vi "updateTCPEvnts.vi"(8 "error in (no error)":errorcluster, 11 "MonoCommunicator in":refnum<class "MonoCommunicator.lvclass">) -> (0 "error out":errorcluster, 3 "MonoCommunicator out":refnum<class "MonoCommunicator.lvclass">)   [LabVIEW 2016, in "MonoCommunicator.lvclass"]
uses:
  MonoCommunicator.lvclass
  MonoCommunicator.lvclass/MonoCommunicator.ctl
  MonoPubSubData/MonoPubSubData.lvclass/MonoPubSubData.ctl
  ts_labview_tcp/TCPCommunicator/TCPCommunicator.lvclass/TCPCommunicator.ctl
  ts_labview_tcp/TCPComEvents/TCPComEvents.lvclass/TCPComEvents.ctl
  ts_labview_tcp/TCPServer/TCPServer.lvclass
  C:/Users/ComputerAdmin/Documents/ts_monochromator_windows/ts_labview_tcp/TCPCommunicator/TCPCommunicator.lvclass
  MonoPubSubData/MonoPubSubData.lvclass
  ts_labview_tcp/TCPComEvents/TCPComEvents.lvclass
  ts_labview_tcp/TCPCommunicator/TCPCommunicator.lvclass
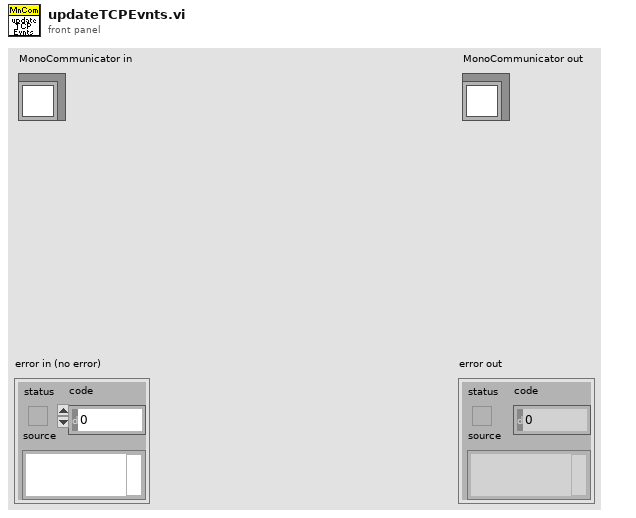
[diagram p1: front panel]
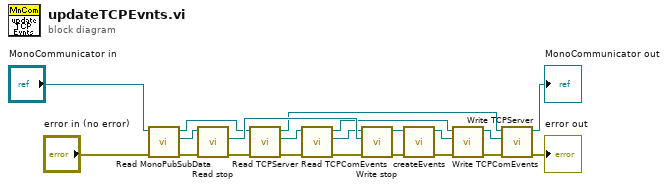
[diagram p0: block diagram]
diagram:
  n1 = call "Read MonoPubSubData.vi"("error in (no error)"="error in (no error)", "MonoCommunicator in"="MonoCommunicator in") -> ("error out"=w7:errorcluster, "MonoPubSubData.lvclass"=w19:refnum<class "MonoPubSubData.lvclass">, "MonoCommunicator out"=w17:refnum<class "MonoCommunicator.lvclass">)  [unwired: 7 in]
  n2 = call "Read stop.vi"("error in (no error)"=w7, "MonoPubSubData in"=w19) -> ("error out"=w8:errorcluster, "stop"=w18:refnum<user-event>)  [unwired: 7 in, 1 out]
  n3 = call "Read TCPServer.vi"("error in (no error)"=w8, "MonoCommunicator in"=w17) -> ("error out"=w16:errorcluster, "TCPServer.lvclass"=w15:refnum<class "TCPServer.lvclass">, "MonoCommunicator out"=w14:refnum<class "MonoCommunicator.lvclass">)  [unwired: 7 in]
  n4 = call "Read TCPComEvents.vi"("error in (no error)"=w16, "TCPCommunicator in"=w15) -> ("error out"=w5:errorcluster, "TCPComEvents.lvclass"=w12:refnum<class "TCPComEvents.lvclass">, "TCPCommunicator out"=w13:refnum<class "TCPServer.lvclass">)  [unwired: 7 in]
  n5 = call "Write stop.vi"("error in (no error)"=w5, "stop"=w18, "TCPComEvents in"=w12) -> ("error out"=w3:errorcluster, "TCPComEvents out"=w4:refnum<class "TCPComEvents.lvclass">)  [unwired: 7 in]
  n6 = call "createEvents.vi"("error in (no error)"=w3, "TCPComEvents in"=w4) -> ("error out"=w2:errorcluster, "TCPComEvents out"=w1:refnum<class "TCPComEvents.lvclass">)  [unwired: 8 in]
  n7 = call "Write TCPComEvents.vi"("error in (no error)"=w2, "TCPComEvents.lvclass"=w1, "TCPCommunicator in"=w13) -> ("error out"=w11:errorcluster, "TCPCommunicator out"=w21:refnum<class "TCPServer.lvclass">)  [unwired: 7 in]
  n8 = call "Write TCPServer.vi"("error in (no error)"=w11, "TCPServer.lvclass"=w21, "MonoCommunicator in"=w14) -> ("error out"=→"error out":errorcluster, "MonoCommunicator out"=→"MonoCommunicator out":refnum<class "MonoCommunicator.lvclass">)  [unwired: 7 in]
